vi "StopDAQ.vi"(8 "error in":errorcluster, 11 "Refnum in":refnum<k21>) -> (0 "error out":errorcluster)   [LabVIEW 2017, in "AODControl.lvlib"]
uses:
  AODControl.lvlib
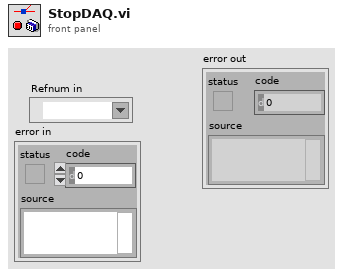
[diagram p1: front panel]
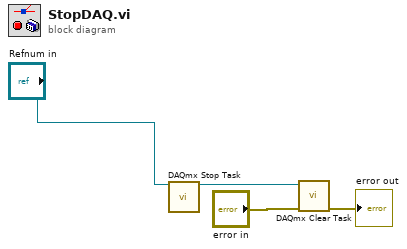
[diagram p0: block diagram]
diagram:
  n1 = call <vilib>:"DAQmx Stop Task.vi"("task/channels in"="Refnum in") -> ("task out"=w1:refnum<k21>)  [unwired: 13 in, 1 out]
  n2 = call <vilib>:"DAQmx Clear Task.vi"("task in"=w1, "error in"="error in") -> ("error out"=→"error out":errorcluster)  [unwired: 13 in]
